vi "Parse-IPv4.vi"(11 "IPv4 Packet (in)":u8[](array[numeric])=[69, 0, 0, 60, 12, 166, 0, 0, 128, 1, 169, 57, 192, 168, 1, 200, 192, 168, 1, 201, 8, 0, 77, 77, 0, 1, 0, 14, 97, 98, 99, 100, 101, 102, 103, 104, 105, 106, 107, 108, 109, 110, 111, 112, 113, 114, 115, 116, 117, 118, 119, 97, 98, 99, 100, 101, 102, 103, 104, 105] format="%02x") -> (0 "Destination IP":u8[](array[numeric])=[192, 168, 1, 201], 1 "Source IP":u8[](array[numeric])=[192, 168, 1, 200], 2 "Header\nChecksum\nOk?":bool=TRUE, 3 "Header":T1={"Version"=4, "Header Length"=20, "Total Length"=60, "More Fragments"=FALSE, "Don't Fragment"=FALSE, "Fragment Offset"=0, "TTL"=128, "Header Checksum"=43321, "Identification"=3238, "Protocol"=1} {"Header Checksum" format="%04x"}, 4 "IPv4 Payload":u8[](array[numeric])=[8, 0, 77, 77, 0, 1, 0, 14, 97, 98, 99, 100, 101, 102, 103, 104, 105, 106, 107, 108, 109, 110, 111, 112, 113, 114, 115, 116, 117, 118, 119, 97, 98, 99, 100, 101, 102, 103, 104, 105] format="%02x")   [LabVIEW 2017]
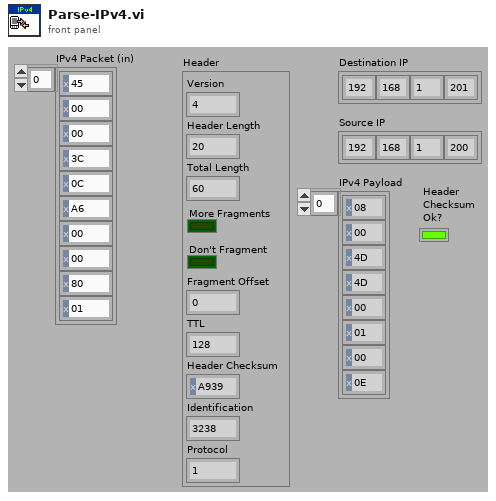
[diagram p1: front panel]
types:
  T1 = cluster{"Version":u8, "Header Length":u8, "Total Length":u16, "More Fragments":bool, "Don't Fragment":bool, "Fragment Offset":u16, "TTL":u8, "Header Checksum":u16, "Identification":u16, "Protocol":u8}
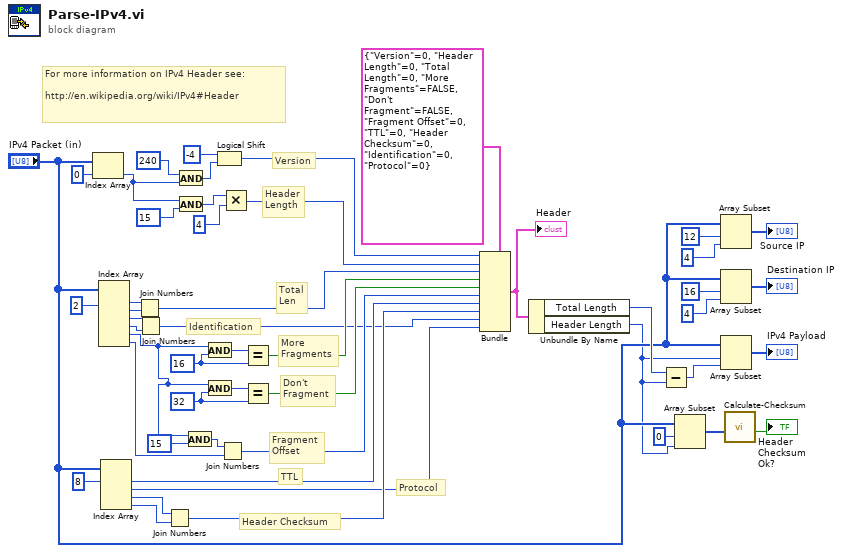
[diagram p0: block diagram]
diagram:
  w42 = u8 32 ("y")
  w40 = u8 16 ("y")
  # "Identification"
  # "Header Checksum"
  # "Protocol"
  # "TTL"
  # "Don't\nFragment"
  # "More\nFragments"
  # "Fragment\nOffset"
  # "Total\nLen"
  # "Header\nLength"
  # "Version"
  # "For more information on IPv4 Header see:\n\nhttp://en.wikipedia.org/wiki/IPv4#Header"
  n1 = Index Array(array="IPv4 Packet (in)", index=0) -> (element=w8:u8)
  n2 = Index Array(array="IPv4 Packet (in)", index #1=2 ("index")) -> (element #1=w22:u8, element #2=w21:u8, element #3=w23:u8, element #4=w24:u8, element #5=w44:u8, element #6=w25:u8)  [unwired: 5 in]
  n3 = Index Array(array="IPv4 Packet (in)", index #1=8 ("index")) -> (element #1=w47:u8, element #2=w14:u8, element #3=w29:u8, element #4=w30:u8)  [unwired: 3 in]
  n4 = Join Numbers(hi=w22, lo=w21) -> ((hi.lo)=w5:u16)
  n5 = Join Numbers(hi=w23, lo=w24) -> ((hi.lo)=w7:u16)
  n6 = Join Numbers(hi=w29, lo=w30) -> ((hi.lo)=w48:u16)
  n7 = And(x=u8 240 ("y"), y=w8) -> (x .and. y?=w11:u8)
  n8 = And(x=w8, y=u8 15) -> (x .and. y?=w18:u8)
  n9 = And(x=w44, y=u8 15) -> (x .and. y?=w27:u8)
  n10 = And(x=w44, y=w40) -> (x .and. y?=w39:u8)
  n11 = And(x=w44, y=w42) -> (x .and. y?=w43:u8)
  n12 = Logical Shift(y=i8 -4, x=w11) -> (x << y=w10:u8)
  n13 = Join Numbers(hi=w27, lo=w25) -> ((hi.lo)=w46:u16)
  n14 = Multiply(x=w18, y=u8 4) -> (x*y=w4:u8)
  n15 = Equal?(x=w39, y=w40) -> (x = y?=w41:bool)
  n16 = Equal?(x=w43, y=w42) -> (x = y?=w45:bool)
  n17 = Bundle(cluster=T1 {"Version"=0, "Header Length"=0, "Total Length"=0, "More Fragments"=FALSE, "Don't Fragment"=FALSE, "Fragment Offset"=0, "TTL"=0, "Header Checksum"=0, "Identification"=0, "Protocol"=0} ("Header"), "Version"=w10, "Header Length"=w4, "Total Length"=w5, "More Fragments"=w41, "Don't Fragment"=w45, "Fragment Offset"=w46, "TTL"=w47, "Header Checksum"=w48, "Identification"=w7, "Protocol"=w14) -> (w6:T1)
  "Header" <- w6
  n18 = Unbundle By Name(w6) -> ("Total Length"=w3:u16, "Header Length"=w1:u8)
  n19 = Subtract(x=w3, y=w1) -> (x-y=w38:u16)
  n20 = Array Subset(array="IPv4 Packet (in)", index=0, length=w1) -> (w50:u8[])
  n21 = Array Subset(array="IPv4 Packet (in)", index=12, length=4) -> (→"Source IP":u8[])
  n22 = Array Subset(array="IPv4 Packet (in)", index=16, length=4) -> (→"Destination IP":u8[])
  n23 = Array Subset(array="IPv4 Packet (in)", index=w1, length=w38) -> (→"IPv4 Payload":u8[])
  n24 = call "Calculate-Checksum.vi"("Array"=w50) -> ("Checksum OK?"=→"Header\nChecksum\nOk?":bool)  [unwired: 9 in, 1 out]
